vi "APDM Get Single Opal Data.vi"(0 "APDM Context":T5={"APDM Context ID"=0, "Gyro Mode"="", "Log Data"=FALSE, "Log File"=refnum, "Gyro Record Log"=refnum, "Gyro CMD Log"=refnum, "L Opal SN"=0, "R Opal SN"=0, "Access Point ID"=0, "Left Gyro Sim Data"=path "C:/Users/jfalesi/Desktop/CP FES Walking Code/Original/Ahad Vi/CP Code/Offline data/TD_7_Raw_R.txt", "Right Gyro Sim Data"=path "C:/Users/jfalesi/Desktop/CP FES Walking Code/Original/Ahad Vi/CP Code/Offline data/TD_7_Raw_R.txt", "Sampling Rate"=0.0, "Gyro Sim Time Array"=[], "Missed Gyro Count"=0.0}, 1 "Left or Right":T4="Left", 2 "Sim Gyro Cluster":T1) -> (4 "Data Log Item":T2, 5 "APDM Context":T5={"APDM Context ID"=0, "Gyro Mode"="", "Log Data"=FALSE, "Log File"=refnum, "Gyro Record Log"=refnum, "Gyro CMD Log"=refnum, "L Opal SN"=0, "R Opal SN"=0, "Access Point ID"=0, "Left Gyro Sim Data"=path "C:/Users/jfalesi/Desktop/CP FES Walking Code/Original/Ahad Vi/CP Code/Offline data/TD_7_Raw_R.txt", "Right Gyro Sim Data"=path "C:/Users/jfalesi/Desktop/CP FES Walking Code/Original/Ahad Vi/CP Code/Offline data/TD_7_Raw_R.txt", "Sampling Rate"=0.0, "Gyro Sim Time Array"=[], "Missed Gyro Count"=0.0}, 6 "Data from Gyro":T3, 7 "Cmd Log String":string)   [LabVIEW 2019]
uses:
  Controls/APDM Context Cluster.ctl
  Archive/CP_FES_Walking_w_stim_on_off.llb/Left_Right_Control.ctl
  Controls/Data From Gyro.ctl
  Controls/APDM Record.ctl
  <vilib>/Utility/file.llb/Read Delimited Spreadsheet (DBL).vi
panel:
  out "output cluster":T1
  out "Sim Gyro Line #":i32
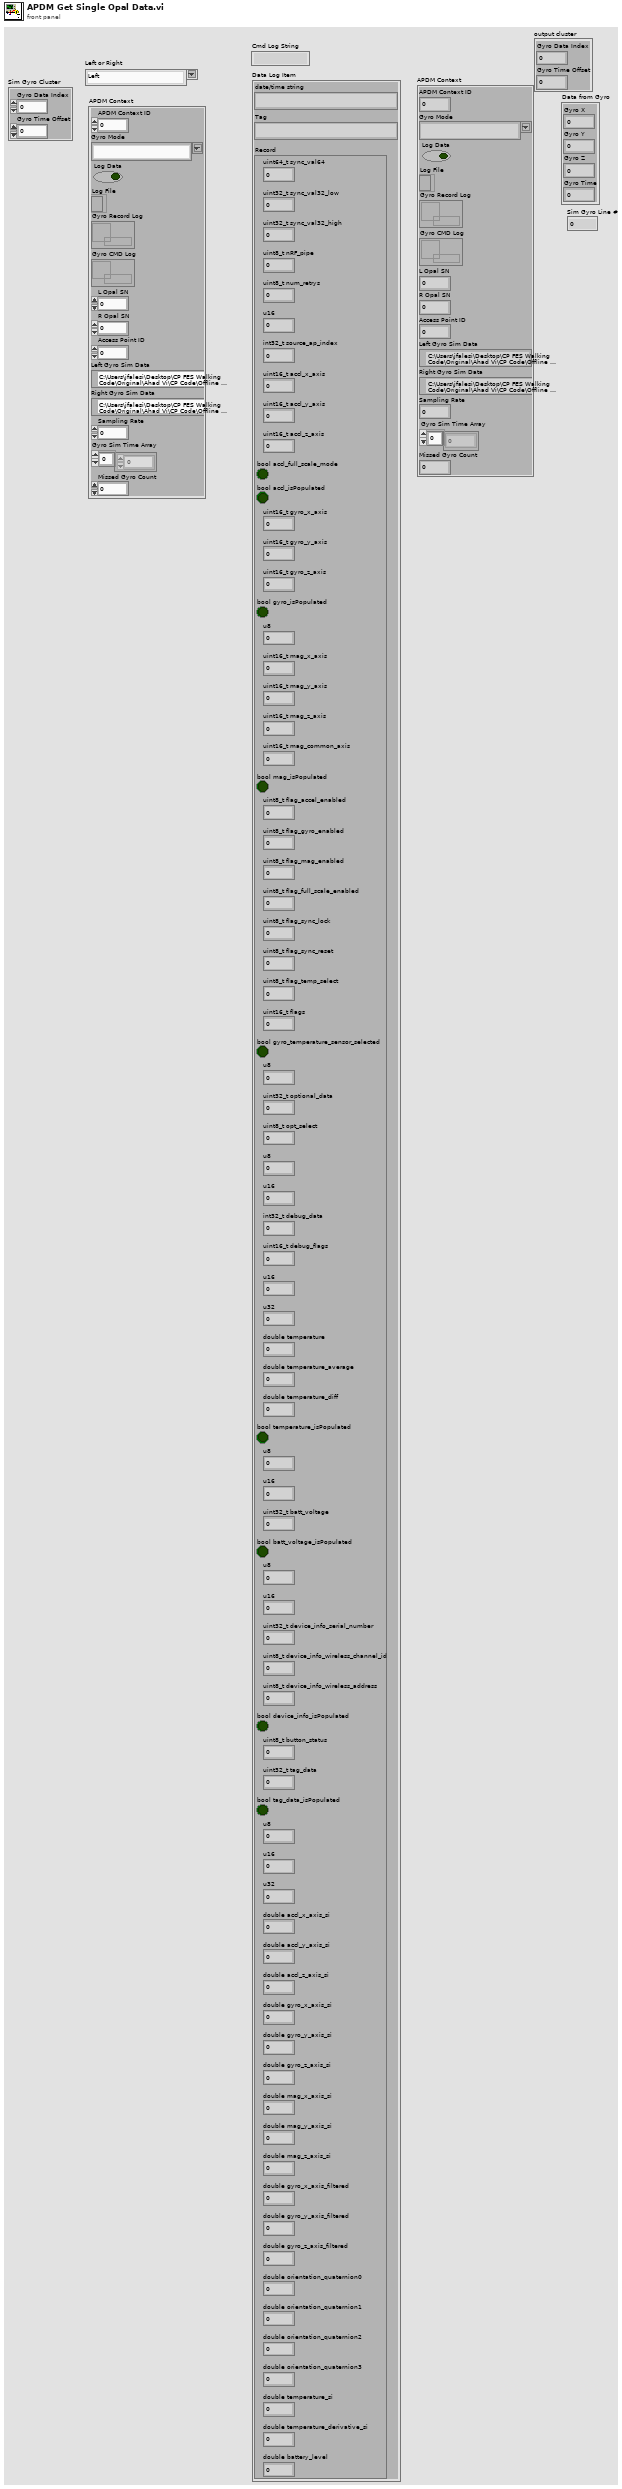
[diagram p1: front panel]
types:
  T1 = cluster{"Gyro Data Index":i32, "Gyro Time Offset":dbl}
  T2 = cluster{"date/time string":string, "Tag":string, "Record":cluster{"uint64_t sync_val64":u64, "uint32_t sync_val32_low":u32, "uint32_t sync_val32_high":u32, "uint8_t nRF_pipe":u8, "uint8_t num_retrys":u8, "u16":u16, "int32_t source_ap_index":i32, "uint16_t accl_x_axis":u16, "uint16_t accl_y_axis":u16, "uint16_t accl_z_axis":u16, "bool accl_full_scale_mode":bool, "bool accl_isPopulated":bool, "uint16_t gyro_x_axis":u16, "uint16_t gyro_y_axis":u16, "uint16_t gyro_z_axis":u16, "bool gyro_isPopulated":bool, "u8":u8, "uint16_t mag_x_axis":u16, "uint16_t mag_y_axis":u16, "uint16_t mag_z_axis":u16, "uint16_t mag_common_axis":u16, "bool mag_isPopulated":bool, "uint8_t flag_accel_enabled":u8, "uint8_t flag_gyro_enabled":u8, "uint8_t flag_mag_enabled":u8, "uint8_t flag_full_scale_enabled":u8, "uint8_t flag_sync_lock":u8, "uint8_t flag_sync_reset":u8, "uint8_t flag_temp_select":u8, "uint16_t flags":u16, "bool gyro_temperature_sensor_selected":bool, "u8":u8, "uint32_t optional_data":u32, "uint8_t opt_select":u8, "u8":u8, "u16":u16, "int32_t debug_data":i32, "uint16_t debug_flags":u16, "u16":u16, "u32":u32, "double temperature":dbl, "double temperature_average":dbl, "double temperature_diff":dbl, "bool temperature_isPopulated":bool, "u8":u8, "u16":u16, "uint32_t batt_voltage":u32, "bool batt_voltage_isPopulated":bool, "u8":u8, "u16":u16, "uint32_t device_info_serial_number":u32, "uint8_t device_info_wireless_channel_id":u8, "uint8_t device_info_wireless_address":u8, "bool device_info_isPopulated":bool, "uint8_t button_status":u8, "uint32_t tag_data":u32, "bool tag_data_isPopulated":bool, "u8":u8, "u16":u16, "u32":u32, "double accl_x_axis_si":dbl, "double accl_y_axis_si":dbl, "double accl_z_axis_si":dbl, "double gyro_x_axis_si":dbl, "double gyro_y_axis_si":dbl, "double gyro_z_axis_si":dbl, "double mag_x_axis_si":dbl, "double mag_y_axis_si":dbl, "double mag_z_axis_si":dbl, "double gyro_x_axis_filtered":dbl, "double gyro_y_axis_filtered":dbl, "double gyro_z_axis_filtered":dbl, "double orientation_quaternion0":dbl, "double orientation_quaternion1":dbl, "double orientation_quaternion2":dbl, "double orientation_quaternion3":dbl, "double temperature_si":dbl, "double temperature_derivative_si":dbl, "double battery_level":dbl}}
  T3 = typedef "Data From Gyro.ctl" = cluster{"Gyro X":dbl, "Gyro Y":dbl, "Gyro Z":dbl, "Gyro Time":dbl}
  T4 = typedef "Left_Right_Control.ctl" = string
  T5 = typedef "APDM Context Cluster.ctl" = cluster{"APDM Context ID":u32, "Gyro Mode":string, "Log Data":bool, "Log File":refnum<file>, "Gyro Record Log":refnum<queue>, "Gyro CMD Log":refnum<queue>, "L Opal SN":u32, "R Opal SN":u32, "Access Point ID":u32, "Left Gyro Sim Data":path, "Right Gyro Sim Data":path, "Sampling Rate":dbl, "Gyro Sim Time Array":dbl[], "Missed Gyro Count":dbl}
  T6 = typedef "APDM Record.ctl" = cluster{"uint64_t sync_val64":u64, "uint32_t sync_val32_low":u32, "uint32_t sync_val32_high":u32, "uint8_t nRF_pipe":u8, "uint8_t num_retrys":u8, "u16":u16, "int32_t source_ap_index":i32, "uint16_t accl_x_axis":u16, "uint16_t accl_y_axis":u16, "uint16_t accl_z_axis":u16, "bool accl_full_scale_mode":bool, "bool accl_isPopulated":bool, "uint16_t gyro_x_axis":u16, "uint16_t gyro_y_axis":u16, "uint16_t gyro_z_axis":u16, "bool gyro_isPopulated":bool, "u8":u8, "uint16_t mag_x_axis":u16, "uint16_t mag_y_axis":u16, "uint16_t mag_z_axis":u16, "uint16_t mag_common_axis":u16, "bool mag_isPopulated":bool, "uint8_t flag_accel_enabled":u8, "uint8_t flag_gyro_enabled":u8, "uint8_t flag_mag_enabled":u8, "uint8_t flag_full_scale_enabled":u8, "uint8_t flag_sync_lock":u8, "uint8_t flag_sync_reset":u8, "uint8_t flag_temp_select":u8, "uint16_t flags":u16, "bool gyro_temperature_sensor_selected":bool, "u8":u8, "uint32_t optional_data":u32, "uint8_t opt_select":u8, "u8":u8, "u16":u16, "int32_t debug_data":i32, "uint16_t debug_flags":u16, "u16":u16, "u32":u32, "double temperature":dbl, "double temperature_average":dbl, "double temperature_diff":dbl, "bool temperature_isPopulated":bool, "u8":u8, "u16":u16, "uint32_t batt_voltage":u32, "bool batt_voltage_isPopulated":bool, "u8":u8, "u16":u16, "uint32_t device_info_serial_number":u32, "uint8_t device_info_wireless_channel_id":u8, "uint8_t device_info_wireless_address":u8, "bool device_info_isPopulated":bool, "uint8_t button_status":u8, "uint32_t tag_data":u32, "bool tag_data_isPopulated":bool, "u8":u8, "u16":u16, "u32":u32, "double accl_x_axis_si":dbl, "double accl_y_axis_si":dbl, "double accl_z_axis_si":dbl, "double gyro_x_axis_si":dbl, "double gyro_y_axis_si":dbl, "double gyro_z_axis_si":dbl, "double mag_x_axis_si":dbl, "double mag_y_axis_si":dbl, "double mag_z_axis_si":dbl, "double gyro_x_axis_filtered":dbl, "double gyro_y_axis_filtered":dbl, "double gyro_z_axis_filtered":dbl, "double orientation_quaternion0":dbl, "double orientation_quaternion1":dbl, "double orientation_quaternion2":dbl, "double orientation_quaternion3":dbl, "double temperature_si":dbl, "double temperature_derivative_si":dbl, "double battery_level":dbl}
  T7 = typedef "Sim Gyro Record.ctl" = cluster{"uint64_t sync_val64":u64, "uint32_t sync_val32_low":u32, "uint32_t sync_val32_high":u32, "uint8_t nRF_pipe":u8, "uint8_t num_retrys":u8, "u16":u16, "int32_t source_ap_index":i32, "uint16_t accl_x_axis":u16, "uint16_t accl_y_axis":u16, "uint16_t accl_z_axis":u16, "bool accl_full_scale_mode":bool, "bool accl_isPopulated":bool, "uint16_t gyro_x_axis":u16, "uint16_t gyro_y_axis":u16, "uint16_t gyro_z_axis":u16, "bool gyro_isPopulated":bool, "u8":u8, "uint16_t mag_x_axis":u16, "uint16_t mag_y_axis":u16, "uint16_t mag_z_axis":u16, "uint16_t mag_common_axis":u16, "bool mag_isPopulated":bool, "uint8_t flag_accel_enabled":u8, "uint8_t flag_gyro_enabled":u8, "uint8_t flag_mag_enabled":u8, "uint8_t flag_full_scale_enabled":u8, "uint8_t flag_sync_lock":u8, "uint8_t flag_sync_reset":u8, "uint8_t flag_temp_select":u8, "uint16_t flags":u16, "bool gyro_temperature_sensor_selected":bool, "u8":u8, "uint32_t optional_data":u32, "uint8_t opt_select":u8, "u8":u8, "u16":u16, "int32_t debug_data":i32, "uint16_t debug_flags":u16, "u16":u16, "u32":u32, "double temperature":dbl, "double temperature_average":dbl, "double temperature_diff":dbl, "bool temperature_isPopulated":bool, "u8":u8, "u16":u16, "uint32_t batt_voltage":u32, "bool batt_voltage_isPopulated":bool, "u8":u8, "u16":u16, "uint32_t device_info_serial_number":u32, "uint8_t device_info_wireless_channel_id":u8, "uint8_t device_info_wireless_address":u8, "bool device_info_isPopulated":bool, "uint8_t button_status":u8, "uint32_t tag_data":u32, "bool tag_data_isPopulated":bool, "u8":u8, "u16":u16, "u32":u32, "double accl_x_axis_si":dbl, "double accl_y_axis_si":dbl, "double accl_z_axis_si":dbl, "double gyro_x_axis_si":dbl, "double gyro_y_axis_si":dbl, "double gyro_z_axis_si":dbl, "double mag_x_axis_si":dbl, "double mag_y_axis_si":dbl, "double mag_z_axis_si":dbl, "double gyro_x_axis_filtered":dbl, "double gyro_y_axis_filtered":dbl, "double gyro_z_axis_filtered":dbl, "double orientation_quaternion0":dbl, "double orientation_quaternion1":dbl, "double orientation_quaternion2":dbl, "double orientation_quaternion3":dbl, "double temperature_si":dbl, "double temperature_derivative_si":dbl, "double battery_level":dbl}
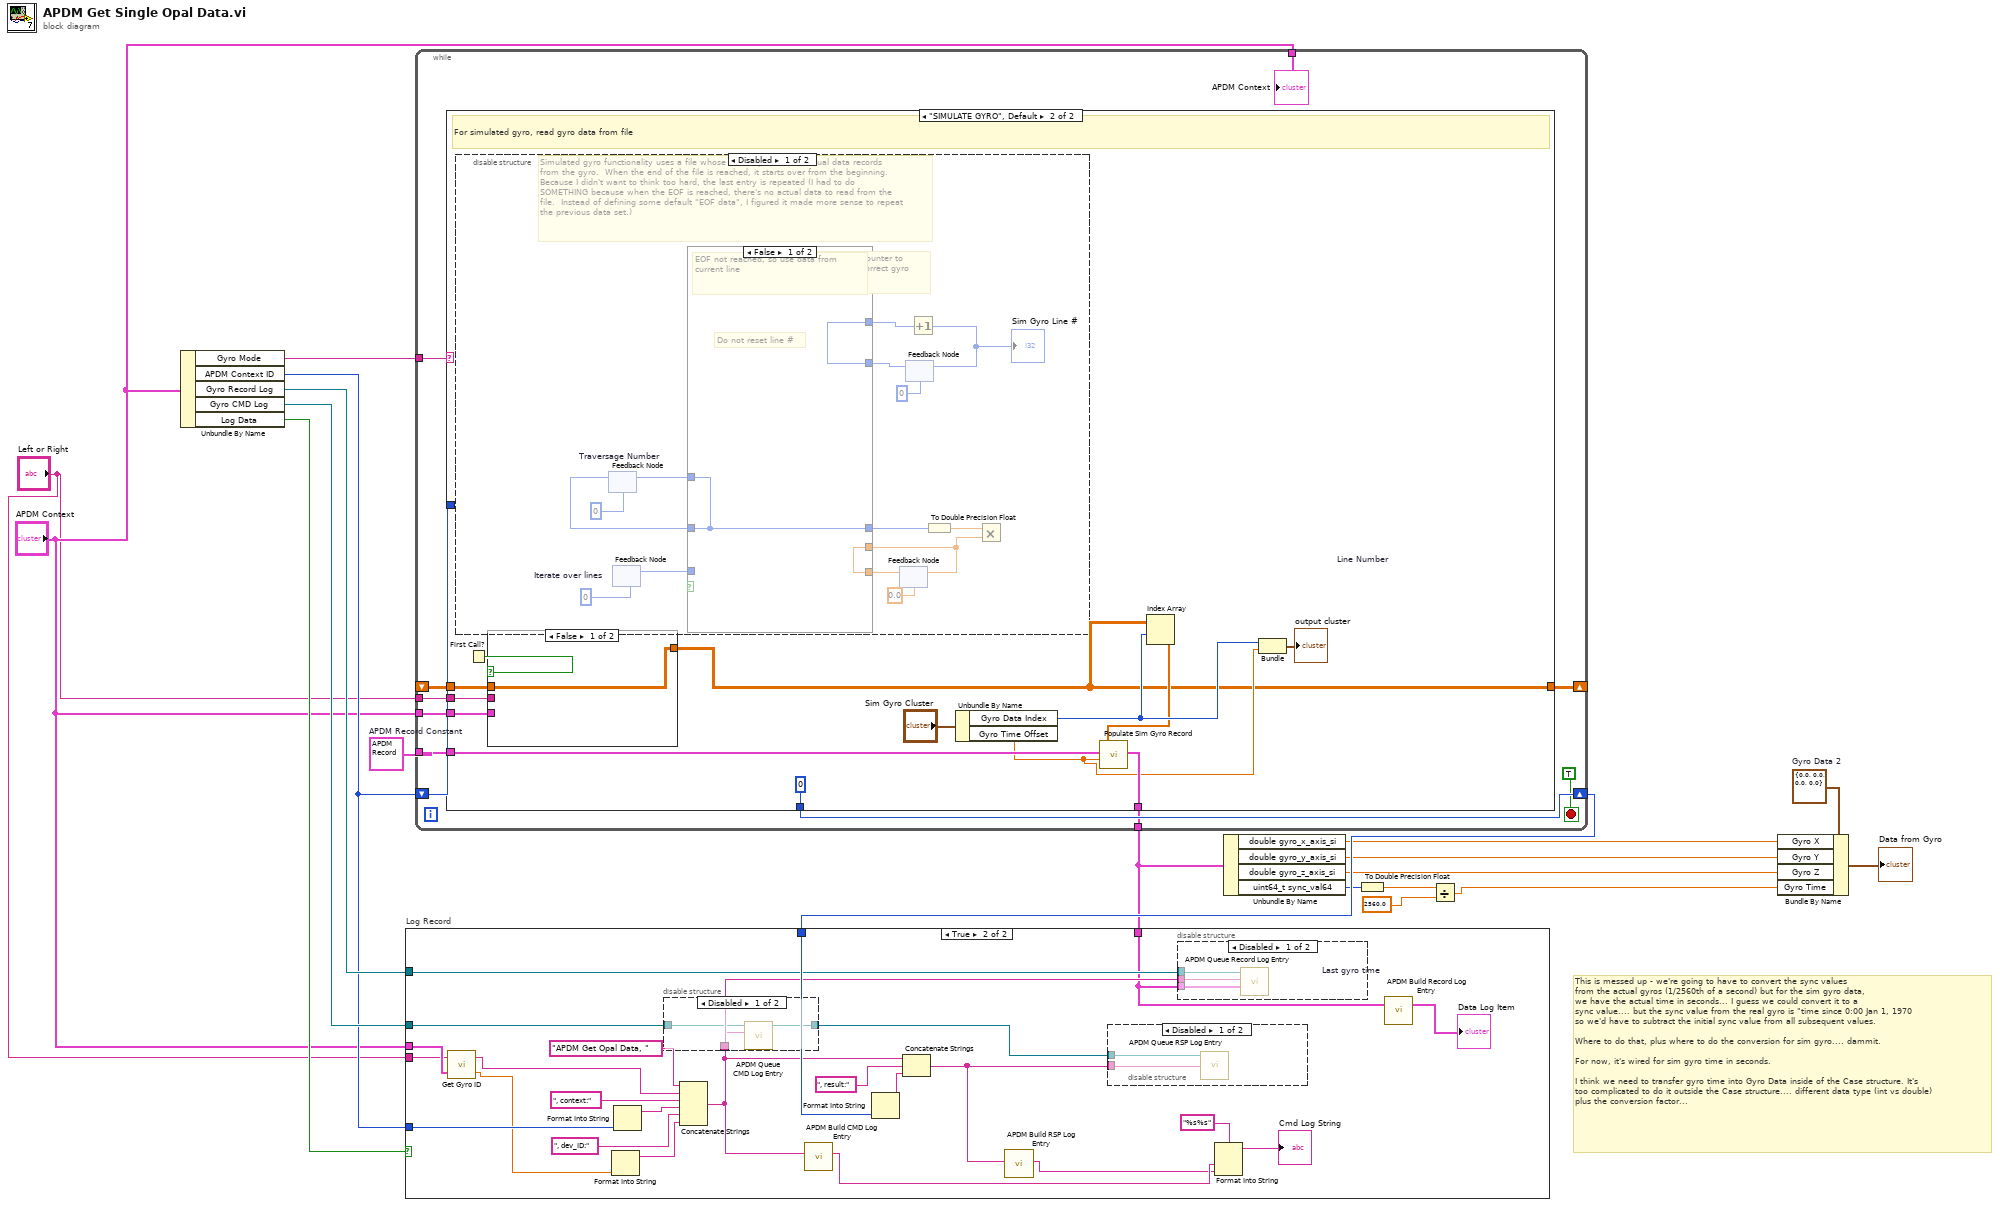
[diagram p0: block diagram]
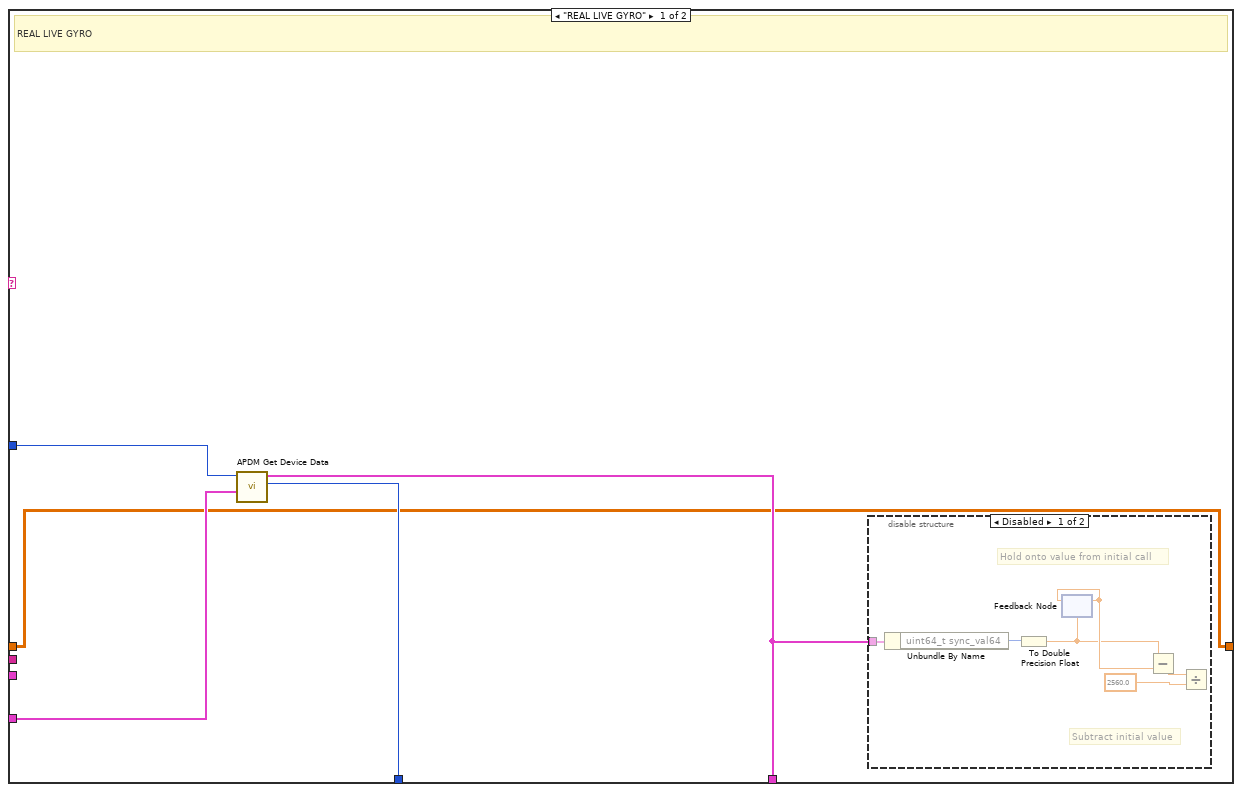
[diagram p2: hidden frame]
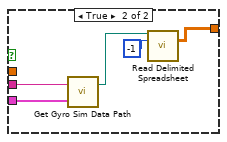
[diagram p4: hidden frame]
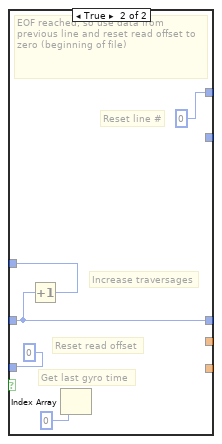
[diagram p5: hidden frame]
diagram:
  w8 = T3 {"Gyro X"=0.0, "Gyro Y"=0.0, "Gyro Z"=0.0, "Gyro Time"=0.0}  # Gyro Data 2
  w13 = T6 {"uint64_t sync_val64"=0, "uint32_t sync_val32_low"=0, "uint32_t sync_val32_high"=0, "uint8_t nRF_pipe"=0, "uint8_t num_retrys"=0, "u16"=0, "int32_t source_ap_index"=0, "uint16_t accl_x_axis"=0, "uint16_t accl_y_axis"=0, "uint16_t accl_z_axis"=0, "bool accl_full_scale_mode"=FALSE, "bool accl_isPopulated"=FALSE, "uint16_t gyro_x_axis"=0, "uint16_t gyro_y_axis"=0, "uint16_t gyro_z_axis"=0, "bool gyro_isPopulated"=FALSE, "u8"=0, "uint16_t mag_x_axis"=0, "uint16_t mag_y_axis"=0, "uint16_t mag_z_axis"=0, "uint16_t mag_common_axis"=0, "bool mag_isPopulated"=FALSE, "uint8_t flag_accel_enabled"=0, "uint8_t flag_gyro_enabled"=0, "uint8_t flag_mag_enabled"=0, "uint8_t flag_full_scale_enabled"=0, "uint8_t flag_sync_lock"=0, "uint8_t flag_sync_reset"=0, "uint8_t flag_temp_select"=0, "uint16_t flags"=0, "bool gyro_temperature_sensor_selected"=FALSE, "u8"=0, "uint32_t optional_data"=0, "uint8_t opt_select"=0, "u8"=0, "u16"=0, "int32_t debug_data"=0, "uint16_t debug_flags"=0, "u16"=0, "u32"=0, "double temperature"=0.0, "double temperature_average"=0.0, "double temperature_diff"=0.0, "bool temperature_isPopulated"=FALSE, "u8"=0, "u16"=0, "uint32_t batt_voltage"=0, "bool batt_voltage_isPopulated"=FALSE, "u8"=0, "u16"=0, "uint32_t device_info_serial_number"=0, "uint8_t device_info_wireless_channel_id"=0, "uint8_t device_info_wireless_address"=0, "bool device_info_isPopulated"=FALSE, "uint8_t button_status"=0, "uint32_t tag_data"=0, "bool tag_data_isPopulated"=FALSE, "u8"=0, "u16"=0, "u32"=0, "double accl_x_axis_si"=0.0, "double accl_y_axis_si"=0.0, "double accl_z_axis_si"=0.0, "double gyro_x_axis_si"=0.0, "double gyro_y_axis_si"=0.0, "double gyro_z_axis_si"=0.0, "double mag_x_axis_si"=0.0, "double mag_y_axis_si"=0.0, "double mag_z_axis_si"=0.0, "double gyro_x_axis_filtered"=0.0, "double gyro_y_axis_filtered"=0.0, "double gyro_z_axis_filtered"=0.0, "double orientation_quaternion0"=0.0, "double orientation_quaternion1"=0.0, "double orientation_quaternion2"=0.0, "double orientation_quaternion3"=0.0, "double temperature_si"=0.0, "double temperature_derivative_si"=0.0, "double battery_level"=0.0}  # APDM Record Constant
  # "This is messed up - we're going to have to convert the sync values \nfrom the actual gyros (1/2560th of a second) but for the sim gyro data,\nwe have the actual time in seconds... I guess we could convert it to a \nsync value.... but the sync value from the real gyro is \"time since 0:00 Jan 1, 1970\nso we'd have to subtract the initial sync value from all subsequent values.\n\nWhere to do that, plus where to do the conversion for sim gyro.... dammit.\n\nFor now, it's wired for sim gyro time in seconds.\n\nI think we need to transfer gyro time into Gyro Data inside of the Case structure. It's\ntoo complicated to do it outside the Case structure.... different data type (int vs double)\nplus the conversion factor..."
  n1 = Unbundle By Name("APDM Context") -> ("Gyro Mode"=w18:string, "APDM Context ID"=w14:u32, "Gyro Record Log"=w17:refnum<queue>, "Gyro CMD Log"=w16:refnum<queue>, "Log Data"=w15:bool)
  n2 = while {
    tunnel: w18 -> [w29]
    tunnel: w13 -> [w27]
    tunnel: "APDM Context" -> [w26]
    tunnel: [w25] -> w7
    shift-right: [w30] -> w19
    shift-left: w14 -> [w28]
    shift-right: [w24] -> _
    shift-left: _ -> [w23]
    tunnel: "APDM Context" -> [w21]
    tunnel: "Left or Right" -> [w20]
    stop <- TRUE stop-if-true
    n3 = case shown="\"SIMULATE GYRO\", Default" w29 {
      tunnel: w27 -> [w35 w54]
      tunnel: w28 -> [w34 _]
      tunnel: [w33 0] -> w30
      tunnel: [w32 w52] -> w25
      tunnel: [w31 w46] -> w24
      tunnel: w23 -> [w31 w45]
      tunnel: w21 -> [_ w43]
      tunnel: w20 -> [_ w42]
      frame "REAL LIVE GYRO" {
        # "REAL LIVE GYRO"
        n4 = call "APDM Get Device Data.vi"("APDM Record Constant"=w35, "APDM Context ID"=w34) -> ("return type"=w33:u32, "Record"=w32:T6)  [unwired: 4 in]
        n5 = disable-structure shown="Disabled" {
          disable-tunnel: w32 -> [w41 _]
          frame Disabled {
            # "Subtract initial value"
            # "Hold onto value from initial call"
            n6 = Unbundle By Name(w41) -> ("uint64_t sync_val64"=w40:u64)
            n7 = To Double Precision Float(number=w40) -> (double precision float=w36:dbl)
            n8 = feedback #1(w36) -> (w37:dbl)
            n9 = feedback-in #1(w37) -> ()
            n10 = Subtract(x=w36, y=w37) -> (x-y=w38:dbl)
            n11 = Divide(x=w38, y=2560.0) -> ()  [unwired: 1 out]
          }
          frame Enabled {
          }
        }
      }
      frame "SIMULATE GYRO", Default {
        # "For simulated gyro, read gyro data from file"
        n12 = disable-structure shown="Disabled" {
          frame Disabled {
            # "Need a cycle counter to\ncompute the correct gyro\ntime"
            # "Simulated gyro functionality uses a file whose lines represent individual data records from the gyro.  When the end of the file is reached, it starts over from the beginning.  Because I didn't want to think too hard, the last entry is repeated (I had to do SOMETHING because when the EOF is reached, there's no actual data to read from the file.  Instead of defining some default \"EOF data\", I figured it made more sense to repeat the previous data set.)"
            n13 = feedback #2 "Traversage Number"(0) -> (w71:i32)
            n14 = feedback #3 "Iterate over lines"(0) -> ()  [unwired: 1 in]
            n15 = feedback #4 "Last gyro time"(0.0) -> (w62:dbl)
            n16 = feedback #5 "Line Number"(0) -> (w65:i32)
            n17 = case shown="False" {
              selector: _ -> [_ _]
              tunnel: [_ 0] -> w74
              tunnel: w71 -> [w77 w81]
              tunnel: [w77 w82] -> w70
              tunnel: [w77 w81] -> w69
              tunnel: w65 -> [w76 _]
              tunnel: [w76 0] -> w64
              tunnel: w62 -> [w75 _]
              tunnel: [w75 _] -> w61
              frame False {
                # "Do not reset line #"
                # "EOF not reached, so use data from current line"
              }
              frame True {
                # "Get last gyro time"
                # "Reset read offset"
                # "Increase traversages"
                # "Reset line #"
                # "EOF reached, so use data from previous line and reset read offset to zero (beginning of file)"
                n18 = Increment(x=w81) -> (x+1=w82:i32)
                n19 = Index Array(index=0) -> ()  [unwired: 1 in, 1 out]
              }
            }
            n20 = feedback-in #2(w70) -> ()
            n21 = feedback-in #3(w74) -> ()
            n22 = feedback-in #4(w61) -> ()
            n23 = Increment(x=w64) -> (x+1=w66:i32)
            "Sim Gyro Line #" <- w66
            n24 = feedback-in #5(w66) -> ()
            n25 = To Double Precision Float(number=w69) -> (double precision float=w67:dbl)
            n26 = Multiply(x=w67, y=w61) -> ()  [unwired: 1 out]
          }
          frame Enabled {
          }
        }
        n27 = First Call?() -> (First Call?: T/F=w44:bool)
        n28 = case shown="False" w44 {
          tunnel: [w55 w60] -> w46
          tunnel: w45 -> [w55 _]
          tunnel: w43 -> [_ w58]
          tunnel: w42 -> [_ w57]
          frame False {
          }
          frame True {
            n29 = call "Get Gyro Sim Data Path.vi"("APDM Context"=w58, "Left or Right"=w57) -> ("Gyro Sim Data Path"=w56:path)  [unwired: 1 in]
            n30 = call-poly <vilib>:"Read Delimited Spreadsheet.vi"("file path (dialog if empty)"=w56, "number of rows (all:-1)"=-1) -> ("all rows"=w60:dbl[][])  [unwired: 8 in, 5 out]
          }
        }
        n31 = Unbundle By Name("Sim Gyro Cluster") -> ("Gyro Data Index"=w49:i32, "Gyro Time Offset"=w50:dbl)
        n32 = Index Array(array=w46, index (row)=w49) -> (element=w47:dbl[])  [unwired: 1 in]
        n33 = call "Populate Sim Gyro Record.vi"("Time Offset"=w50, "Empty Sim Gyro Record"=w54, "Sim Gyro Data"=w47) -> ("Sim Gyro Record"=w52:T7)  [unwired: 4 in]
        n34 = Bundle("Gyro Data Index"=w49, "Gyro Time Offset"=w50) -> (→"output cluster":T1)  [unwired: 1 in]
      }
    }
    "APDM Context" <- w26
  }
  n35 = case "Log Record" shown="True" w15 {
    tunnel: w16 -> [_ w106]
    tunnel: w19 -> [_ w103]
    tunnel: w14 -> [_ w104]
    tunnel: w7 -> [_ w88]
    tunnel: w17 -> [_ w97]
    tunnel: "APDM Context" -> [_ w86]
    tunnel: "Left or Right" -> [_ w85]
    frame False {
    }
    frame True {
      n36 = call "Get Gyro ID.vi"("APDM Context"=w86, "Left or Right"=w85) -> ("Opal SN"=w83:dbl, "L or R"=w84:string)
      n37 = Format Into String(w83) -> (resulting string=w101:string)  [unwired: 3 in, 1 out]
      n38 = Format Into String(w104) -> (resulting string=w96:string)  [unwired: 3 in, 1 out]
      n39 = Concatenate Strings("APDM Get Opal Data, " ("Log Item"), w84, ", context:" ("string"), w96, ", dev_ID:" ("string"), w101) -> (w94:string)
      n40 = disable-structure shown="Disabled" {
        disable-tunnel: w106 -> [w114 _]
        disable-tunnel: [w113 _] -> w98
        disable-tunnel: w94 -> [w112 _]
        frame Disabled {
          n41 = call "APDM Queue CMD Log Entry.vi"("Log Item"=w112, "Gyro Log Queue"=w114) -> ("queue out"=w113:refnum<queue>)  [unwired: 8 in, 1 out]
        }
        frame Enabled {
        }
      }
      n42 = call "APDM Build CMD Log Entry.vi"("Log Item"=w94) -> ("Log Entry"=w91:string)  [unwired: 10 in]
      n43 = Format Into String(w103) -> (resulting string=w100:string)  [unwired: 3 in, 1 out]
      n44 = Concatenate Strings(w94, ", result:" ("string"), w100) -> (w93:string)
      n45 = call "APDM Build RSP Log Entry.vi"("Log Item"=w93) -> ("Log Entry"=w90:string)  [unwired: 10 in]
      n46 = disable-structure shown="Disabled" {
        disable-tunnel: w98 -> [w108 _]
        disable-tunnel: w93 -> [w107 _]
        frame Disabled {
          n47 = call "APDM Queue RSP Log Entry.vi"("Log Item"=w107, "Gyro Log Queue"=w108) -> ()  [unwired: 8 in, 2 out]
        }
        frame Enabled {
        }
      }
      n48 = disable-structure shown="Disabled" {
        disable-tunnel: w97 -> [w111 _]
        disable-tunnel: w88 -> [w110 _]
        disable-tunnel: w94 -> [w109 _]
        frame Disabled {
          n49 = call "APDM Queue Record Log Entry.vi"("Record"=w110, "Tag"=w109, "Gyro Record Log Queue"=w111) -> ()  [unwired: 7 in, 2 out]
        }
        frame Enabled {
        }
      }
      n50 = Format Into String(format string="%s%s", w91, w90) -> (resulting string=→"Cmd Log String":string)  [unwired: 2 in, 1 out]
      n51 = call "APDM Build Record Log Entry.vi"("Record"=w88) -> ("output cluster"=→"Data Log Item":T2)  [unwired: 2 in]
    }
  }
  n52 = Unbundle By Name(w7) -> ("double gyro_x_axis_si"=w12:dbl, "double gyro_y_axis_si"=w11:dbl, "double gyro_z_axis_si"=w10:dbl, "uint64_t sync_val64"=w6:u64)
  n53 = To Double Precision Float(number=w6) -> (double precision float=w4:dbl)
  n54 = Divide(x=w4, y=2560.0) -> (x/y=w3:dbl)
  n55 = Bundle By Name(cluster=w8, "Gyro X"=w12, "Gyro Y"=w11, "Gyro Z"=w10, "Gyro Time"=w3) -> (→"Data from Gyro":T3)
